vi "ROI entry-Load and compare Z norm.vi"(8 "error in (no error)":errorcluster, 11 "Old ROI file path":path) -> (0 "error out":errorcluster, 1 "Both Zplane Pockels Values files exist":bool, 2 "Z Norm is Different":bool, 3 "Latest Zplane_Pockels_Values file data (header removed)":dbl[][](array[numeric]), 4 "Older [Z norm]":dbl[](array[numeric]), 5 "Latest [Z norm]":dbl[](array[numeric]), 6 "Older Zplane_Pockels_Values file data (header removed)":dbl[][](array[numeric]))   [LabVIEW 2013]
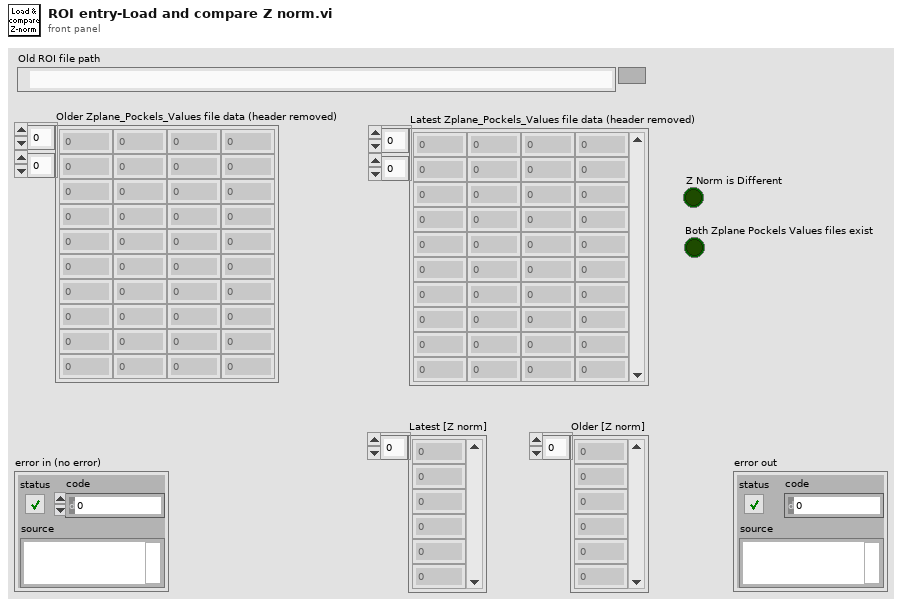
[diagram p1: front panel]
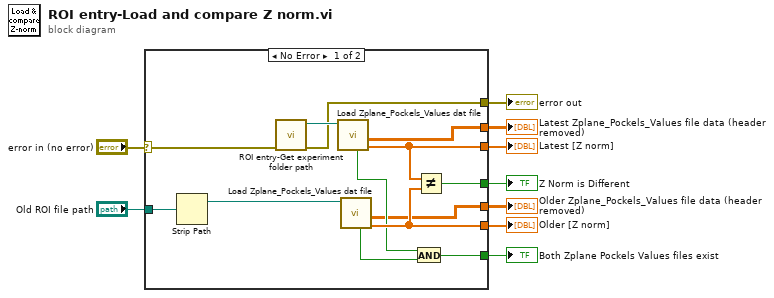
[diagram p0: block diagram]
diagram:
  n1 = case shown="No Error" "error in (no error)" {
    selector: "error in (no error)" -> [w15 w23]
    tunnel: [w21 _] -> w9
    tunnel: [w20 _] -> w8
    tunnel: "Old ROI file path" -> [w18 _]
    tunnel: [w17 _] -> w6
    tunnel: [w16 _] -> w5
    tunnel: [w11 _] -> w4
    tunnel: [w14 w23] -> w2
    tunnel: [w10 _] -> w1
    frame No Error {
      n2 = Strip Path(path=w18) -> (stripped path=w19:path)  [unwired: 1 out]
      n3 = call "ROI entry-Get experiment folder path.vi"("error in (no error)"=w15) -> ("error out"=w14:errorcluster, "Experiment folder path"=w22:path)  [unwired: 9 in]
      n4 = call "Load Zplane_Pockels_Values dat file.vi"("Experiment data folder path"=w22) -> ("[Z norm]"=w17:dbl[], "Zplane_Pockels_Values file data (header removed)"=w21:dbl[][], "Zplane Pockels values file exists"=w12:bool)  [unwired: 5 in, 3 out]
      n5 = call "Load Zplane_Pockels_Values dat file.vi"("Experiment data folder path"=w19) -> ("[Z norm]"=w16:dbl[], "Zplane_Pockels_Values file data (header removed)"=w10:dbl[][], "Zplane Pockels values file exists"=w13:bool)  [unwired: 5 in, 3 out]
      n6 = And(x=w12, y=w13) -> (x .and. y?=w11:bool)
      n7 = Not Equal?(x=w17, y=w16) -> (x != y?=w20:bool)
    }
    frame Error {
    }
  }
  "Latest Zplane_Pockels_Values file data (header removed)" <- w9
  "Z Norm is Different" <- w8
  "Latest [Z norm]" <- w6
  "Older [Z norm]" <- w5
  "Both Zplane Pockels Values files exist" <- w4
  "error out" <- w2
  "Older Zplane_Pockels_Values file data (header removed)" <- w1
